vi "Timer.vi"(7 "TimerAction":T1, 8 "error in (no error)":errorcluster, 11 "Time To Elapse":dbl) -> (0 "error out":errorcluster, 2 "TimeElapsed?":bool, 3 "Elapsed Time":dbl)   [LabVIEW 2017]
doc: "This VI ....."
uses:
  Timer Actions.ctl
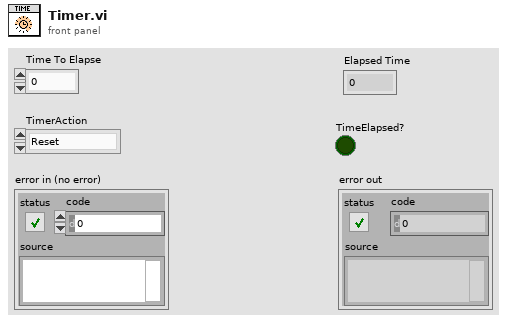
[diagram p1: front panel]
types:
  T1 = typedef "Timer Actions.ctl" = enum16{"Reset", "Check Time"}
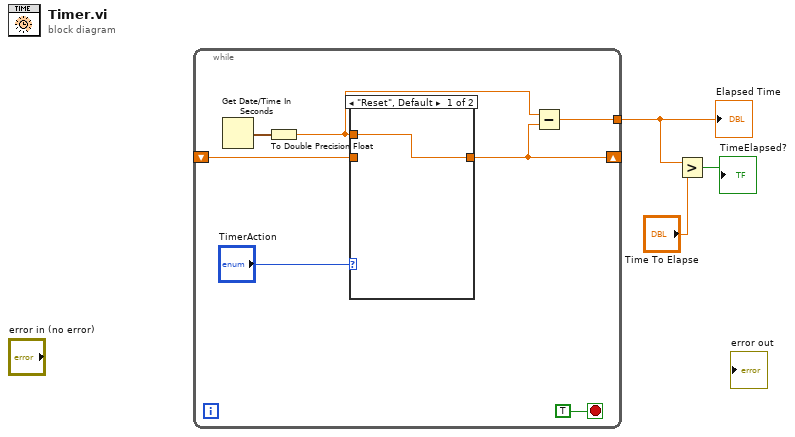
[diagram p0: block diagram]
diagram:
  n1 = while {
    shift-right: [w5] -> _
    shift-left: _ -> [w7]
    tunnel: [w4] -> w3
    stop <- TRUE stop-if-true
    n2 = Get Date/Time In Seconds() -> (seconds since 1Jan1904=w10:timestamp)
    n3 = To Double Precision Float(number=w10) -> (double precision float=w6:dbl)
    n4 = case shown="\"Reset\", Default" "TimerAction" {
      tunnel: w6 -> [w11 _]
      tunnel: [w11 w12] -> w5
      tunnel: w7 -> [_ w12]
      frame "Reset", Default {
      }
      frame "Check Time" {
      }
    }
    n5 = Subtract(x=w6, y=w5) -> (x-y=w4:dbl)
  }
  "Elapsed Time" <- w3
  n6 = Greater?(x=w3, y="Time To Elapse") -> (0:→"TimeElapsed?":bool)
